vi "Determine Battery State.vi"(11 "Voltage":fxp<+/-,24,5>) -> (0 "Low Battery":bool, 1 "Running":bool, 2 "Fully Charged":bool, 3 "Battery State":T1)   [LabVIEW 2015]
doc: "This VI uses a voltage to determine the state of the battery. It returns an enum which shows the battery state as well as a set of boolean values with the same information."
uses:
  Custom Controls/Battery State.ctl
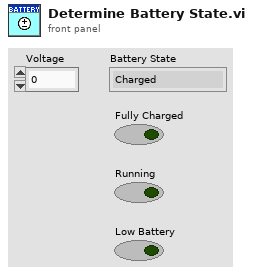
[diagram p1: front panel]
types:
  T1 = typedef "Battery State.ctl" = enum16{"Charged", "Running", "Low Batt"}
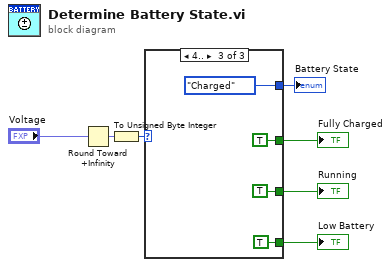
[diagram p0: block diagram]
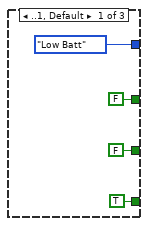
[diagram p2: hidden frame]
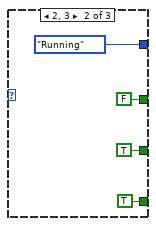
[diagram p3: hidden frame]
diagram:
  n1 = Round Toward +Infinity(x="Voltage") -> (ceil(x): smallest int >= x=w6:fxp<+/-,6,6>)
  n2 = To Unsigned Byte Integer(number=w6) -> (unsigned 8bit integer=w7:u8)
  n3 = case shown="4.." w7 {
    tunnel: [Battery_State."Low Batt" Battery_State."Running" Battery_State."Charged"] -> w4
    tunnel: [FALSE FALSE TRUE] -> w1
    tunnel: [FALSE TRUE TRUE] -> w2
    tunnel: [TRUE TRUE TRUE] -> w3
    frame ..1, Default {
    }
    frame 2, 3 {
    }
    frame 4.. {
    }
  }
  "Battery State" <- w4
  "Low Battery" <- w3
  "Running" <- w2
  "Fully Charged" <- w1
